vi "Configured Acquisition Trigger (Host).vi"() -> ()   [LabVIEW 2021]
doc: "Use this VI as a template to design an application that acquires data using advanced triggering logic from the NI PXIe-5170R/5171R."
uses:
  <instrlib>/_niInstr/Data Trigger/v1/Shared/Public/Level Configuration Trigger When.ctl
  <instrlib>/_niInstr/Data Trigger/v1/Shared/Public/Edge Configuration Trigger Slope.ctl
  <instrlib>/HSAI-RIO/Types/v1/Host/Typedefs/Temp Source.ctl
  <vilib>/FPGAPlugInAG/PXIe-5170R (8CH)/niLvFpga_Open_PXIe-5170R (8CH).vi
  <vilib>/rvi/interface/common/dynamic/niFpgaDynamicAddResources.vi
  <vilib>/FPGAPlugInAG/Dynamic/niLvFpga_Close_Dynamic.vi
  <vilib>/rvi/interface/nirviOpenFPGA/nirviOpenFPGA.xnode
  FPGA Bitfiles/Multirecord_Acquisition_NI_PXIe-5170R_8CH.lvbitx
  <vilib>/rvi/interface/nirviCloseFPGA/nirviCloseFPGA.xnode
  Device Session/Device Session.lvclass
  <instrlib>/HSAI-RIO/Types/v1/Host/niHSAI Types v1 Host.lvlib
  <instrlib>/_niInstr/Data Trigger/v1/Shared/niInstr Data Trigger v1 Shared.lvlib
panel:
  out "actual sample rate":dbl format="%#_6p"
  in  "onboard sample clock rate":dbl(ring)=250000000.0 items=["250 MHz"=250000000.0, "200 MHz"=200000000.0, "150 MHz"=150000000.0]
  in  "impedance":enum8{"Default", "1 mega ohm", "50 ohm"}(ring)
  in  "vertical offset (V)":dbl format="%.2p"
  out "Waveform Graph":T1(graph)
  out "fpga temperature (°C)":dbl(slide)=60.0 scale=0.0..96.0 scale format="%#_6p"
  out "power consumption (W)":dbl(slide)=20.0 scale=0.0..38.25 scale format="%#_6p"
  in  "mode":T2(ring)=enum."High Resolution"
  in  "decimation factor":u16=1
  in  "coupling":enum8{"Default", "DC", "AC"}(ring)
  in  "bandwidth":T3(ring)
  in  "trigger source B":u8
  in  "trigger source A":u8
  in  "pretrigger samples":u64=500
  in  "B":enum32{"Edge", "Level"}(tab)
  in  "hysteresis (%fs)":dbl=0.25
  in  "trigger level (V)":dbl
  in  "trigger slope":T4
  in  "trigger level (V)":dbl
  in  "trigger when":T5
  in  "A":enum32{"Edge", "Level"}(tab)
  in  "hysteresis (%fs)":dbl=0.25
  in  "trigger level (V)":dbl
  in  "trigger slope":T4
  in  "trigger level (V)":dbl
  in  "trigger when":T5
  in  "number of samples":u64=1000
  in  "RIO Device":tag
  in  "channel(s)":string="0,1"
  in  "timeout (ms)":i32=5000
  in  "vertical range (Vpp)":dbl=1.0 format="%.2p"
  out "error out":errorcluster
  in  "stop":bool
  # "RIO Device"
  # "Vertical Settings"
  # "Trigger Settings"
  # "System Monitor"
  # "A"
  # "B"
  # "Acquisition Settings"
  # "Clocking"
  # "DSP"
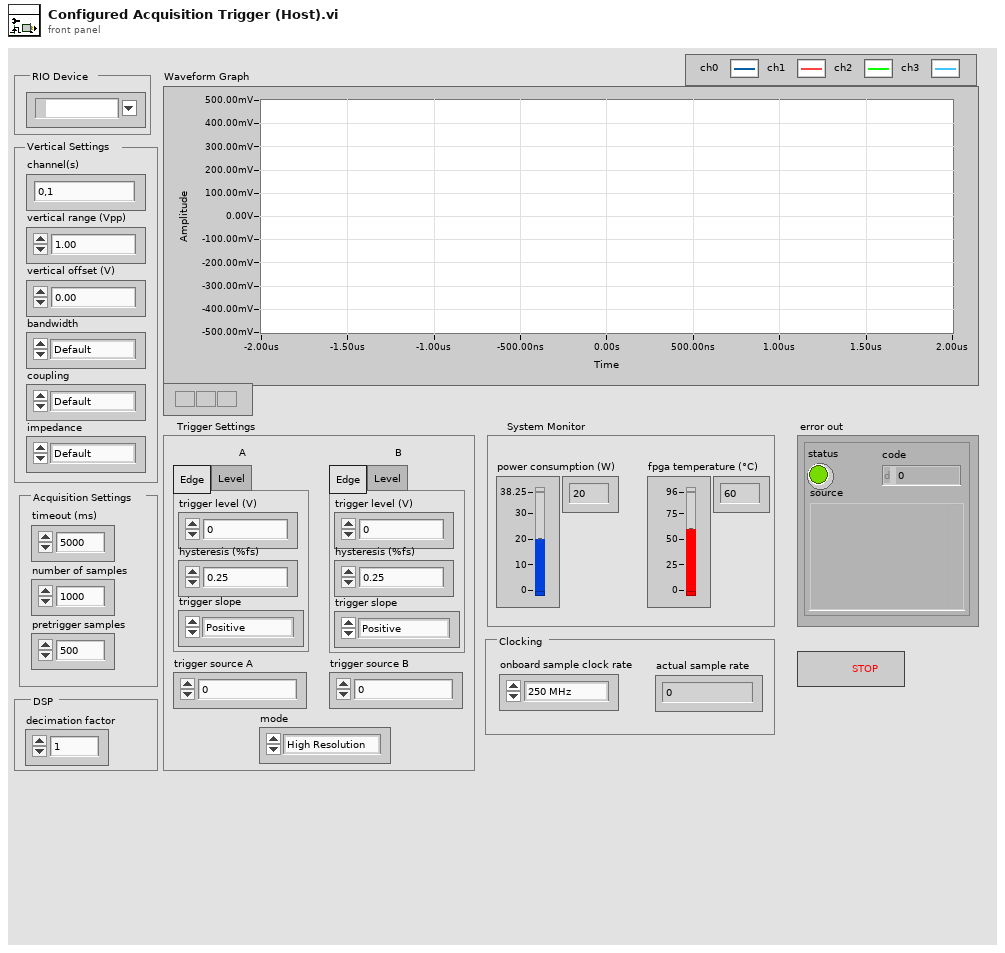
[diagram p1: front panel]
types:
  T1 = cluster{"relativeX":dbl, "sample rate":dbl, "data in":dbl[]}[]
  T2 = enum16{"Immediate", "A", "B", "OR", "AND", "A THEN B", "B THEN A", "High Resolution"}
  T3 = enum8{"Default", "Full Bandwidth", "Anti-alias Filter", "80 MHz FIR Filter", "40 MHz FIR Filter", "20 MHz FIR Filter"}
  T4 = typedef "niInstr Data Trigger v1 Shared.lvlib/Edge Configuration Trigger Slope.ctl" = enum8{"Positive", "Negative"}
  T5 = typedef "niInstr Data Trigger v1 Shared.lvlib/Level Configuration Trigger When.ctl" = enum8{"Trigger Above", "Trigger Below"}
  T6 = typedef "niHSAI Types v1 Host.lvlib/Temp Source.ctl" = enum8{"Device Temperature", "Thermal Shutdown Margin", "FPGA Temperature", "FPGA Temperature Limit"}
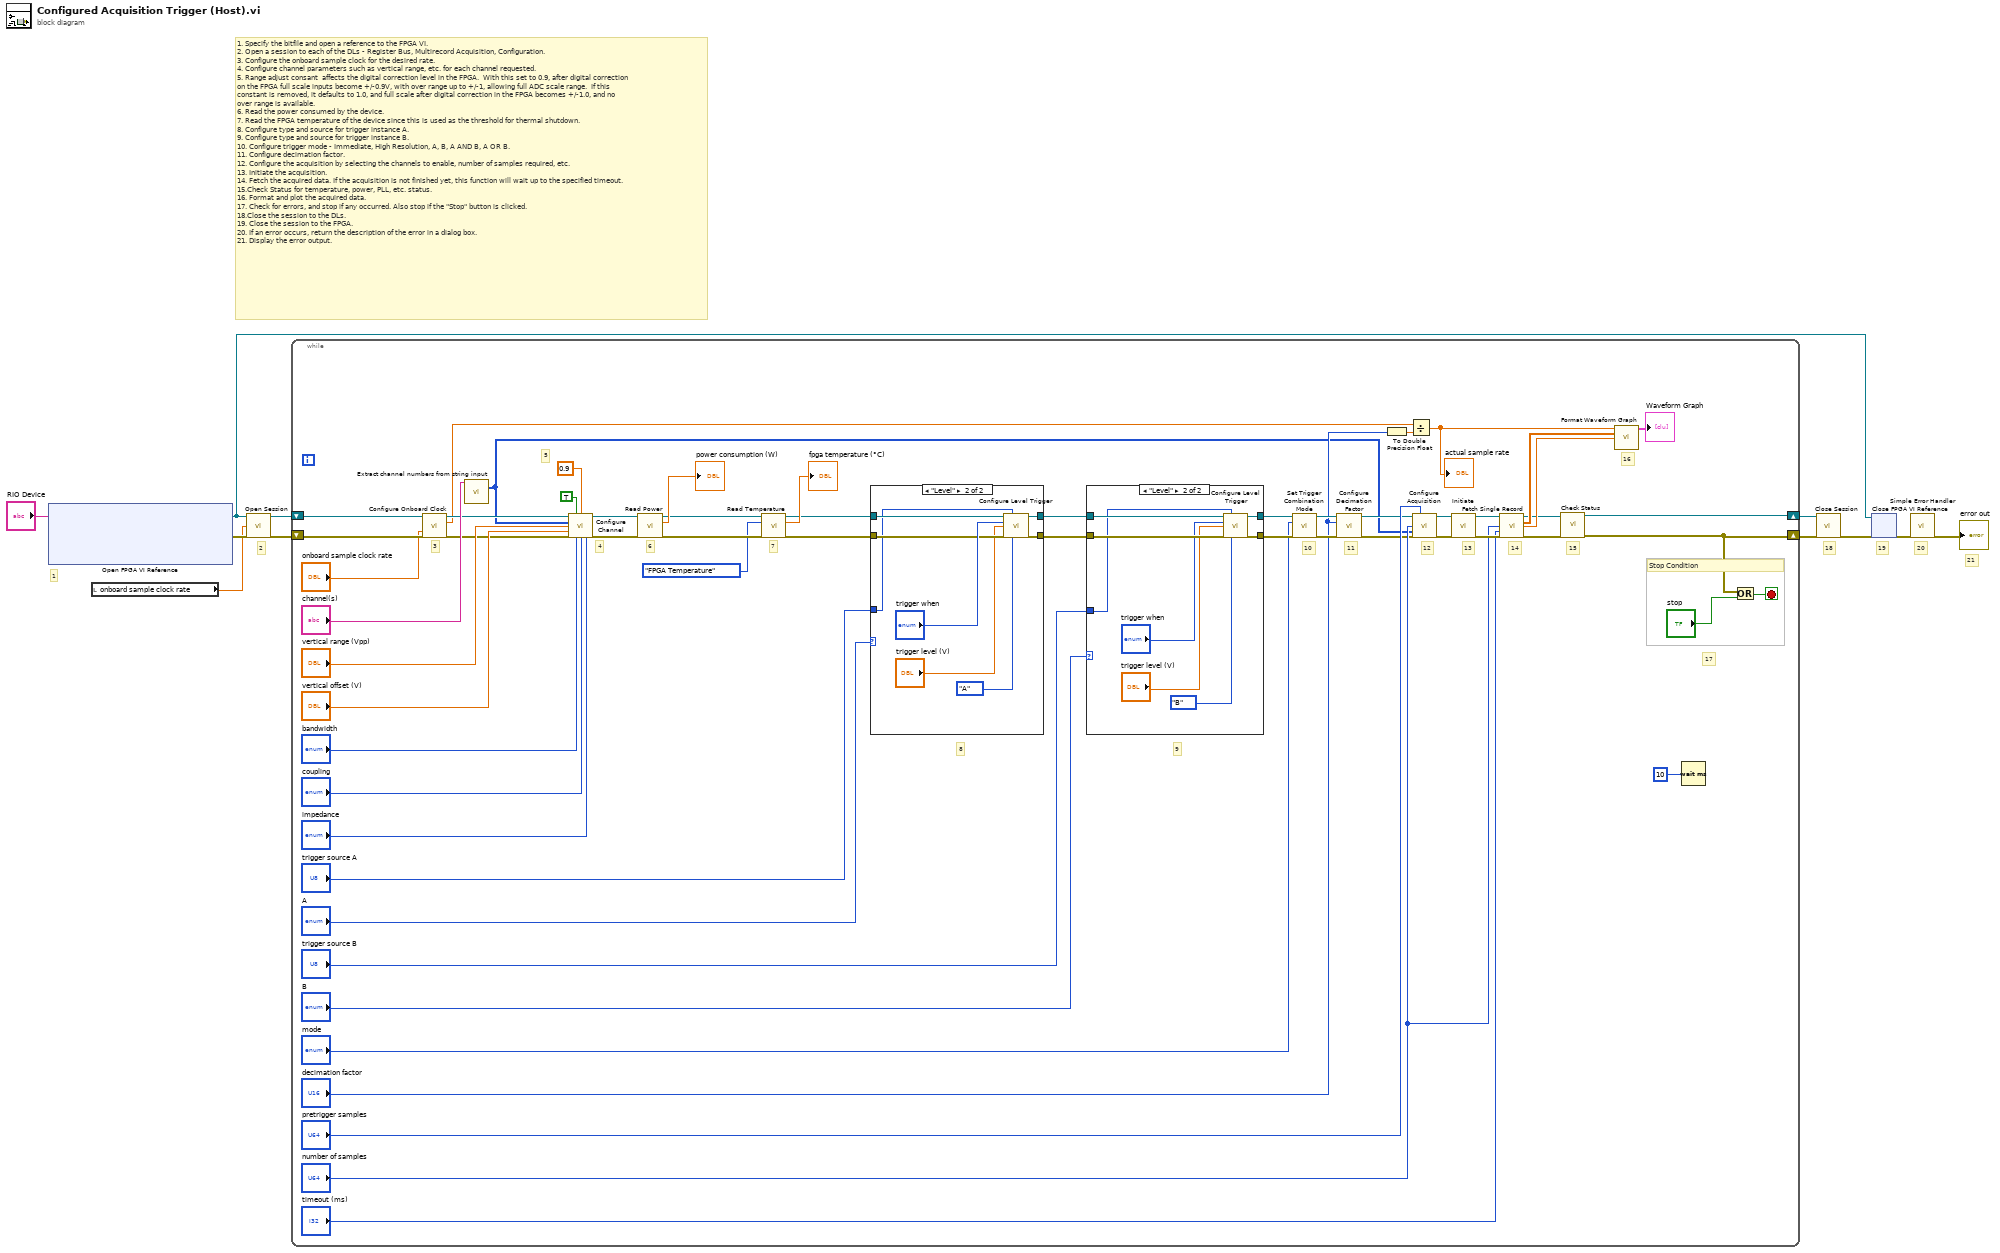
[diagram p0: block diagram]
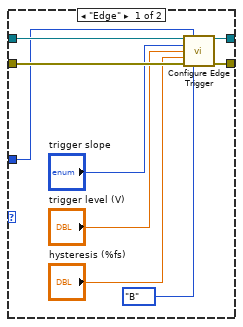
[diagram p2: hidden frame]
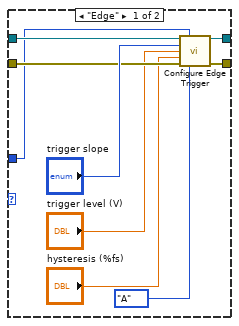
[diagram p3: hidden frame]
diagram:
  # "21"
  # "20"
  # "19"
  # "18"
  # "1. Specify the bitfile and open a reference to the FPGA VI.\n2. Open a session to each of the DLs - Register Bus, Multirecord Acquisition, Configuration.\n3. Configure the onboard sample clock for the desired rate.\n4. Configure channel parameters such as vertical range, etc. for each channel requested.\n5. Range adjust consant  affects the digital correction level in the FPGA.  With this set to 0.9, after digital correction\non the FPGA full scale inputs become +/-0.9V, with over range up to +/-1, allowing full ADC scale range.  If this \nconstant is removed, it defaults to 1.0, and full scale after digital correction in the FPGA becomes +/-1.0, and no\nover range is available.  \n6. Read the power consumed by the device.\n7. Read the FPGA temperature of the device since this is used as the threshold for thermal shutdown.\n8. Configure type and source for trigger instance A.\n9. Configure type and source for trigger instance B.\n10. Configure trigger mode - Immediate, High Resolution, A, B, A AND B, A OR B.\n11. Configure decimation factor.\n12. Configure the acquisition by selecting the channels to enable, number of samples required, etc.\n13. Initiate the acquisition.\n14. Fetch the acquired data. If the acquisition is not finished yet, this function will wait up to the specified timeout.\n15.Check Status for temperature, power, PLL, etc. status. \n16. Format and plot the acquired data.\n17. Check for errors, and stop if any occurred. Also stop if the \"Stop\" button is clicked.\n18.Close the session to the DLs.\n19. Close the session to the FPGA.\n20. If an error occurs, return the description of the error in a dialog box.\n21. Display the error output."
  # "2"
  # "1"
  n1 = xnode "Open FPGA VI Reference"("resource name"="RIO Device") -> ("FPGA VI Reference Out"=w3:refnum<k20>, "error out"=w5:errorcluster)  [unwired: 1 in]
  n2 = local read "onboard sample clock rate"() -> (w1:dbl)
  n3 = call "Open Session.vi"("fpga reference in"=w3, "adc clock rate (Hz)"=w1, "error in"=w5) -> ("device session out"=w9:refnum<class "Device Session.lvclass">, "error out"=w8:errorcluster)  [unwired: 11 in]
  n4 = while {
    shift-right: [w32] -> w11
    shift-left: w8 -> [w44]
    shift-right: [w30] -> w10
    shift-left: w9 -> [w45]
    stop <- w58 stop-if-true
    # "4"
    # "5"
    # "7"
    # "6"
    # "15"
    # "11"
    # "3"
    # "Stop Condition"
    # "17"
    # "16"
    # "10"
    # "9"
    # "8"
    # "14"
    # "13"
    # "12"
    n5 = call "Configure Onboard Clock.vi"("device session in"=w45, "adc clock rate (Hz)"="onboard sample clock rate", "error in"=w44) -> ("device session out"=w43:refnum<class "Device Session.lvclass">, "actual adc clock rate (Hz)"=w35:dbl, "error out"=w42:errorcluster)  [unwired: 9 in, 1 out]
    n6 = call "Extract channel numbers from string input.vi"("channel input"="channel(s)") -> ("array of chans"=w12:u32[])  [unwired: 13 in, 1 out]
    n7 = call "Configure Channel.vi"("device session in"=w43, "enable channel (T)"=TRUE ("enable channel"), "range adjust"=0.9, "channels"=w12, "vertical range (Vpp)"="vertical range (Vpp)", "vertical offset (V)"="vertical offset (V)", "error in"=w42, "bandwidth"="bandwidth", "coupling"="coupling", "impedance"="impedance") -> ("device session out"=w25:refnum<class "Device Session.lvclass">, "error out"=w24:errorcluster)  [unwired: 4 in]
    n8 = call "Read Power.vi"("device session in"=w25, "error in"=w24) -> ("device session out"=w26:refnum<class "Device Session.lvclass">, "power (W)"=→"power consumption (W)":dbl, "error out"=w27:errorcluster)  [unwired: 11 in]
    n9 = call "Read Temperature.vi"("device session in"=w26, "source"=Temp_Source."FPGA Temperature", "error in"=w27) -> ("device session out"=w23:refnum<class "Device Session.lvclass">, "temperature (°C)"=→"fpga temperature (°C)":dbl, "error out"=w22:errorcluster)  [unwired: 10 in]
    n10 = case shown="\"Level\"" "A" {
      tunnel: w22 -> [w92 w100]
      tunnel: w23 -> [w94 w102]
      tunnel: [w90 w99] -> w56
      tunnel: [w91 w98] -> w55
      tunnel: "trigger source A" -> [w86 w95]
      frame "Edge" {
        n11 = call "Configure Edge Trigger.vi"("device session in"=w94, "trigger source"=w86, "trigger slope"="trigger slope", "trigger level (V)"="trigger level (V)", "hysteresis (%fs)"="hysteresis (%fs)", "error in"=w92, "instance"=enum16{"A", "B"}."A") -> ("device session out"=w90:refnum<class "Device Session.lvclass">, "error out"=w91:errorcluster)  [unwired: 7 in]
      }
      frame "Level" {
        n12 = call "Configure Level Trigger.vi"("device session in"=w102, "trigger source"=w95, "trigger when"="trigger when", "trigger level (V)"="trigger level (V)", "error in"=w100, "instance"=enum16{"A", "B"}."A") -> ("device session out"=w99:refnum<class "Device Session.lvclass">, "error out"=w98:errorcluster)  [unwired: 8 in]
      }
    }
    n13 = case shown="\"Level\"" "B" {
      tunnel: w55 -> [w76 w84]
      tunnel: w56 -> [w77 w85]
      tunnel: [w74 w83] -> w53
      tunnel: [w75 w82] -> w52
      tunnel: "trigger source B" -> [w69 w78]
      frame "Edge" {
        n14 = call "Configure Edge Trigger.vi"("device session in"=w77, "trigger source"=w69, "trigger slope"="trigger slope", "trigger level (V)"="trigger level (V)", "hysteresis (%fs)"="hysteresis (%fs)", "error in"=w76, "instance"=enum16{"A", "B"}."B") -> ("device session out"=w74:refnum<class "Device Session.lvclass">, "error out"=w75:errorcluster)  [unwired: 7 in]
      }
      frame "Level" {
        n15 = call "Configure Level Trigger.vi"("device session in"=w85, "trigger source"=w78, "trigger when"="trigger when", "trigger level (V)"="trigger level (V)", "error in"=w84, "instance"=enum16{"A", "B"}."B") -> ("device session out"=w83:refnum<class "Device Session.lvclass">, "error out"=w82:errorcluster)  [unwired: 8 in]
      }
    }
    n16 = call "Set Trigger Combination Mode.vi"("device session in"=w53, "mode"="mode", "error in"=w52) -> ("device session out"=w40:refnum<class "Device Session.lvclass">, "error out"=w39:errorcluster)  [unwired: 11 in]
    n17 = call "Configure Decimation Factor.vi"("device session in"=w40, "decimation factor"="decimation factor", "error in"=w39) -> ("device session out"=w37:refnum<class "Device Session.lvclass">, "error out"=w38:errorcluster)  [unwired: 11 in]
    n18 = To Double Precision Float(number="decimation factor") -> (double precision float=w41:dbl)
    n19 = Divide(x=w35, y=w41) -> (x/y=w14:dbl)
    "actual sample rate" <- w14
    n20 = call "Configure Acquisition.vi"("device session in"=w37, "pretrigger samples"="pretrigger samples", "number of samples"="number of samples", "channels to store"=w12, "error in"=w38) -> ("device session out"=w64:refnum<class "Device Session.lvclass">, "error out"=w67:errorcluster)  [unwired: 8 in, 1 out]
    n21 = call "Initiate.vi"("device session in"=w64, "error in"=w67) -> ("device session out"=w65:refnum<class "Device Session.lvclass">, "error out"=w66:errorcluster)  [unwired: 12 in]
    n22 = call "Fetch Single Record.vi"("device session in"=w65, "number of samples"="number of samples", "timeout (ms)"="timeout (ms)", "error in"=w66) -> ("device session out"=w31:refnum<class "Device Session.lvclass">, "data"=w47:dbl[][], "relativeX (samples)"=w46:dbl, "error out"=w33:errorcluster)  [unwired: 7 in, 1 out]
    n23 = call "Check Status.vi"("device session in"=w31, "error in"=w33) -> ("device session out"=w30:refnum<class "Device Session.lvclass">, "error out"=w32:errorcluster)  [unwired: 12 in]
    n24 = call "Format Waveform Graph.vi"("sample rate (Hz)"=w14, "data in"=w47, "relativeX (samples)"=w46) -> ("waveform out"=→"Waveform Graph":T1)  [unwired: 12 in]
    n25 = Wait (ms)(milliseconds to wait=u32 10) -> ()  [unwired: 1 out]
    n26 = Or(x=w32, y="stop") -> (x .or. y?=w58:bool)
  }
  n27 = call "Close Session.vi"("device session in"=w10, "error in"=w11) -> ("error out"=w4:errorcluster)  [unwired: 13 in]
  n28 = xnode "Close FPGA VI Reference"("FPGA VI Reference In"=w3, "error in"=w4) -> ("error out"=w2:errorcluster)
  n29 = call <vilib>:"Simple Error Handler.vi"("error in (no error)"=w2) -> ("error out"=→"error out":errorcluster)  [unwired: 4 in, 4 out]
